vi "tm_getelectronframe.vi"(8 "error in (no error)":errorcluster, 9 "Frame Index":i32=-1, 10 "Buffer":T1, 11 "Handle in":u32) -> (0 "error out":errorcluster, 2 "Data 16":sgl[][](array[numeric]), 3 "Handle out":u32)   [LabVIEW 2011]
uses:
  tmcamcon.dll
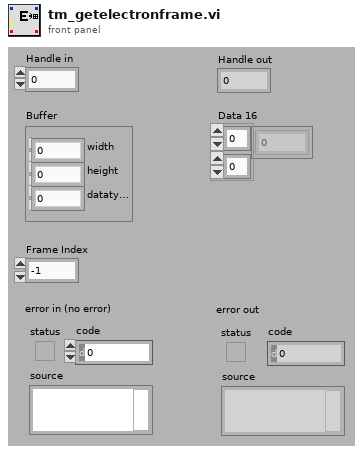
[diagram p1: front panel]
types:
  T1 = cluster{"width":u32, "height":u32, "datatype":u32}
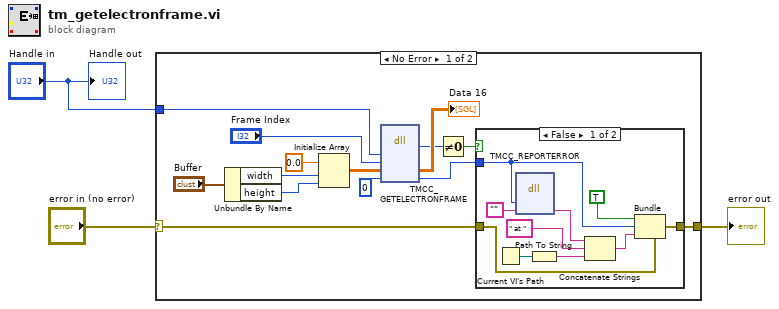
[diagram p0: block diagram]
diagram:
  n1 = case shown="No Error" "error in (no error)" {
    selector: "error in (no error)" -> [w16 w29]
    tunnel: [w15 w29] -> w2
    tunnel: "Handle in" -> [w7 _]
    frame No Error {
      n2 = Unbundle By Name("Buffer") -> ("width"=w11:u32, "height"=w10:u32)
      n3 = Initialize Array(sgl 0.0, w11, w10) -> (w13:sgl[][])
      n4 = dll-call lib="tmcamcon.dll" fn="TMCC_GETELECTRONFRAME"("index"=w7, "frameindex"="Frame Index", "imgarray"=w13, "Erval"=0) -> ("return type"=w4:u32, "imgarray"=→"Data 16":sgl[][], "Erval"=w5:i32)  [unwired: 5 in, 2 out]
      n5 = Not Equal To 0?(x=w4) -> (x != 0?=w17:bool)
      n6 = case shown="False" w17 {
        tunnel: w16 -> [w27 w28]
        tunnel: [w26 w28] -> w15
        tunnel: w5 -> [w20 _]
        frame False {
          n7 = Current VI's Path() -> (path=w25:path)
          n8 = dll-call lib="tmcamcon.dll" fn="TMCC_REPORTERROR"("error"=w20, "buf"="") -> ("buf"=w19:string)  [unwired: 5 in, 2 out]
          n9 = Path To String(path=w25) -> (string=w21:string)
          n10 = Concatenate Strings(w19, " at ", w21) -> (w24:string)
          n11 = Bundle(cluster=w27, "status"=TRUE, "code"=w20, "source"=w24) -> (w26:errorcluster)
        }
        frame True {
        }
      }
    }
    frame Error {
    }
  }
  "error out" <- w2
  "Handle out" <- "Handle in"
